vi "Extract Puzzle Details.vi"(0 "Puzzle Input":string) -> (1 "#Stacks":i32, 2 "Stacks Drawing":string[](array[string]), 3 "Crane Operator Instructions":string[](array[string]))   [LabVIEW 2020, in "AoC 2022.lvlib"]
uses:
  AoC 2022.lvlib
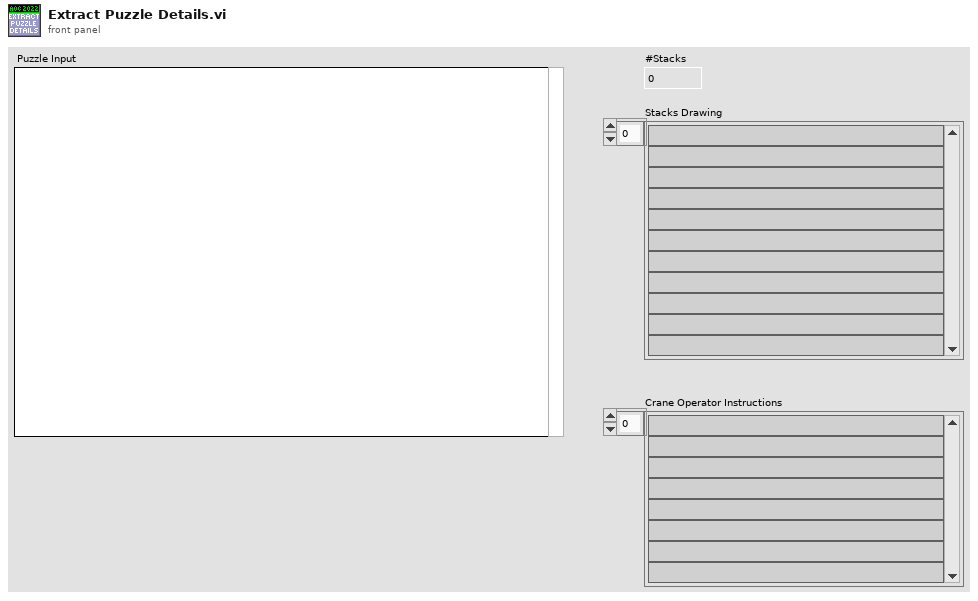
[diagram p1: front panel]
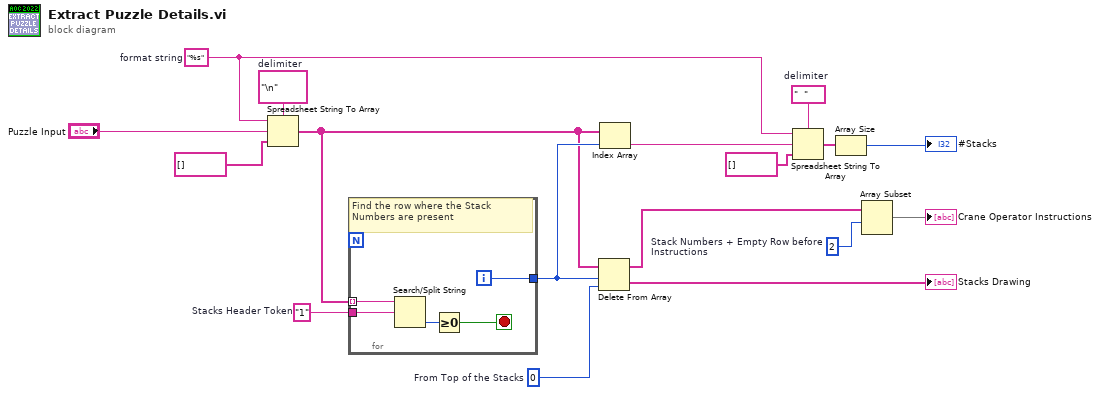
[diagram p0: block diagram]
diagram:
  w2 = "%s"  # format string
  w5 = "\n"  # delimiter
  w17 = 0  # From Top of the Stacks
  w13 = 2  # Stack Numbers + Empty Row before Instructions
  w9 = "1"  # Stacks Header Token
  w6 = "  "  # delimiter
  n1 = Spreadsheet String To Array(delimiter (Tab)=w5, format string=w2, spreadsheet string="Puzzle Input", array type (2D Dbl)=string[] []) -> (array=w3:string[])
  n2 = for {
    tunnel: w3 -> [w22] mode=indexing
    tunnel: w9 -> [w21]
    tunnel: [w18] -> w11
    i -> [w18]
    stop <- w19 stop-if-true
    # "Find the row where the Stack Numbers are present"
    n3 = Search/Split String(string=w22, search string/char (-)=w21) -> (offset of match=w20:i32)  [unwired: 1 in, 2 out]
    n4 = Greater Or Equal To 0?(x=w20) -> (x >= 0?=w19:bool)
  }
  n5 = Delete From Array(array=w3, length=w11, index=w17) -> (deleted portion=→"Stacks Drawing":string[], array with subset deleted=w12:string[])
  n6 = Index Array(array=w3, index=w11) -> (element=w7:string)
  n7 = Spreadsheet String To Array(delimiter (Tab)=w6, format string=w2, spreadsheet string=w7, array type (2D Dbl)=string[] []) -> (array=w10:string[])
  n8 = Array Size(array=w10) -> (size(s)=→"#Stacks":i32)
  n9 = Array Subset(array=w12, index=w13) -> (→"Crane Operator Instructions":string[])  [unwired: 1 in]
